vi "Close.vi"(8 "error in (no error)":errorcluster, 11 "Maxon Encoder in":refnum<class "Maxon Encoder.lvclass">) -> (0 "error out":errorcluster)   [LabVIEW 2019, in "Maxon Encoder.lvclass"]
doc: "Terminates the software connection to the sensor."
uses:
  Maxon Encoder.lvclass
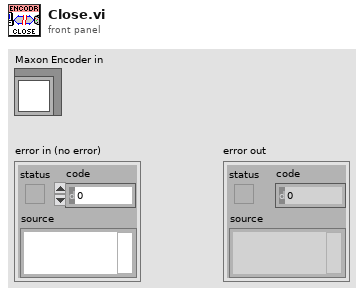
[diagram p1: front panel]
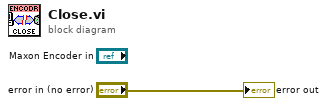
[diagram p0: block diagram]
diagram:
  "error out" <- "error in (no error)"
